vi "Read Data 2.vi"(8 "error in":errorcluster, 11 "Vec3d in":refnum<class "Vec3d.lvclass">) -> (0 "error out":errorcluster, 1 "Z":dbl, 2 "Y":dbl, 3 "X":dbl)   [LabVIEW 2023, in "Vec3d.lvclass"]
uses:
  Vec3d.lvclass
  Vec3d.lvclass/Vec3d.ctl
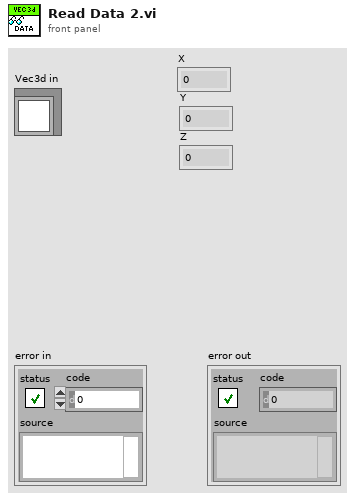
[diagram p1: front panel]
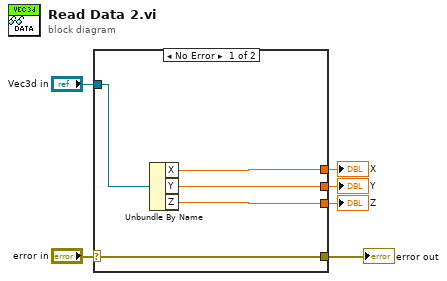
[diagram p0: block diagram]
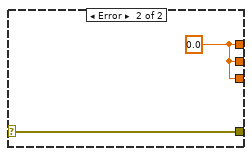
[diagram p2: hidden frame]
diagram:
  n1 = case shown="No Error" "error in" {
    selector: "error in" -> [w11 w13]
    tunnel: [w11 w13] -> w5
    tunnel: "Vec3d in" -> [w10 _]
    tunnel: [w9 w12] -> w3
    tunnel: [w8 w12] -> w2
    tunnel: [w7 w12] -> w1
    frame No Error {
      n2 = Unbundle By Name(w10) -> ("X"=w9:dbl, "Y"=w8:dbl, "Z"=w7:dbl)
    }
    frame Error {
      w12 = 0.0 ("X")
    }
  }
  "error out" <- w5
  "X" <- w3
  "Y" <- w2
  "Z" <- w1
